vi "ErrorModule.vi"(8 "Error In":errorcluster, 11 "CommunicationRefs":T1) -> (0 "Error Out":errorcluster)   [LabVIEW 2015]
uses:
  TypeDefs/CommunicationRefs.ctl
  TypeDefs/MessageCluster.ctl
  <vilib>/event_ctls.llb/usereventprio.ctl
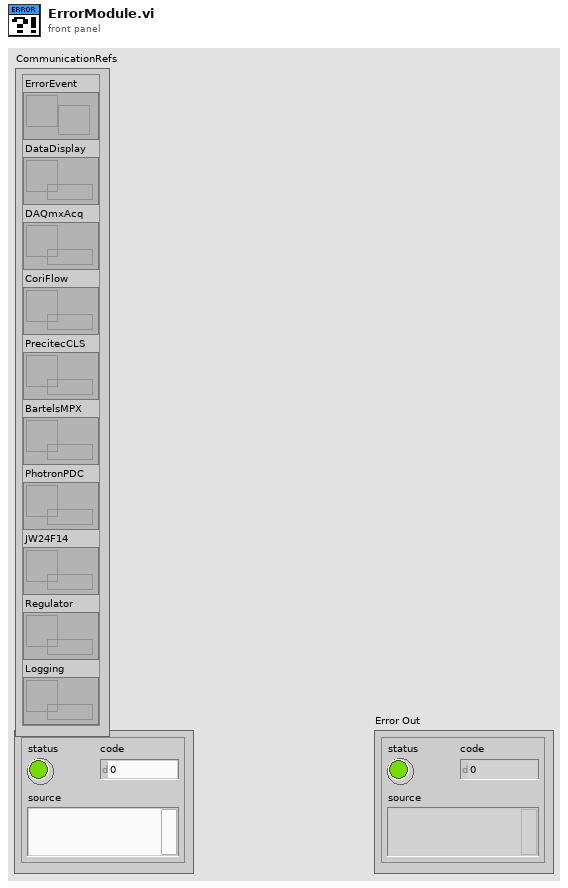
[diagram p1: front panel]
types:
  T1 = typedef "CommunicationRefs.ctl" = cluster{"ErrorEvent":refnum<user-event>, "DataDisplay":refnum<queue>, "DAQmxAcq":refnum<queue>, "CoriFlow":refnum<queue>, "PrecitecCLS":refnum<queue>, "BartelsMPX":refnum<queue>, "PhotronPDC":refnum<queue>, "JW24F14":refnum<queue>, "Regulator":refnum<queue>, "Logging":refnum<queue>}
  T2 = typedef "usereventprio.ctl" = enum32{"high priority", "normal priority"}
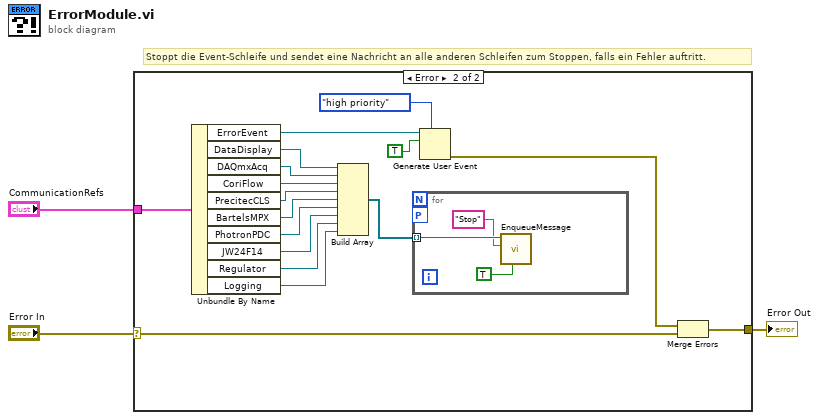
[diagram p0: block diagram]
diagram:
  # "Stoppt die Event-Schleife und sendet eine Nachricht an alle anderen Schleifen zum Stoppen, falls ein Fehler auftritt."
  n1 = case shown="Error" "Error In" {
    selector: "Error In" -> [w4 w10]
    tunnel: [w4 w12] -> w2
    tunnel: "CommunicationRefs" -> [_ w16]
    frame No Error {
    }
    frame Error {
      n2 = Unbundle By Name(w16) -> ("ErrorEvent"=w15:refnum<user-event>, "DataDisplay"=w9:refnum<queue>, "DAQmxAcq"=w17:refnum<queue>, "CoriFlow"=w18:refnum<queue>, "PrecitecCLS"=w19:refnum<queue>, "BartelsMPX"=w20:refnum<queue>, "PhotronPDC"=w8:refnum<queue>, "JW24F14"=w7:refnum<queue>, "Regulator"=w5:refnum<queue>, "Logging"=w6:refnum<queue>)
      n3 = Build Array(w9, w17, w18, w19, w20, w8, w7, w5, w6) -> (w21:refnum<queue>[])
      n4 = for {
        tunnel: w21 -> [w24] mode=indexing
        workers-P: _ -> [_]
        n5 = call "EnqueueMessage.vi"("Priority Message? (F)"=TRUE, "Message"="Stop", "MessageQueue"=w24) -> ()  [unwired: 7 in, 2 out]
      }
      n6 = Generate User Event(priority (normal)=usereventprio."high priority", user event=w15, event data cluster=TRUE ("event data")) -> (error out=w13:errorcluster)  [unwired: 1 in, 1 out]
      n7 = Merge Errors(w13, w10) -> (w12:errorcluster)
    }
  }
  "Error Out" <- w2
